vi "0506_Classificador_de_forma.vi"() -> ()   [LabVIEW 2017]
uses:
  <vilib>/userdefined/High Color/IMAQdx.ctl
  <vilib>/vision/driver/IMAQdx.llb/IMAQdx Acquisition Mode.ctl
  <vilib>/vision/driver/IMAQdx.llb/IMAQdx Buffer Number Mode.ctl
  <vilib>/vision/driver/NI_Vision_Acquisition_Software.lvlib
  <vilib>/vision/NI_Vision_Development_Module.lvlib
panel:
  out "size(s)":i32
  out "Forma":string="Quadrado"
  out "Contorno":cluster{"X":dbl, "Y":dbl}[](graph)
  in  "Operation":T1(ring)=enum."Gradient out"
  in  "Convex Hull":bool=TRUE
  in  "Morphology\nOperation":bool
  in  "Remove small objects":bool=TRUE
  in  "Color Mode":u16(ring) items=["RGB", "HSL", "HSV", "HSI"]
  in  "Red or Hue Range":cluster{"Lower value":sgl, "Upper value":sgl}={"Lower value"=0.0, "Upper value"=255.0} {"Upper value" scale=0.0..255.0; "Lower value" scale=0.0..255.0}
  in  "Green or Sat Range":cluster{"Lower value":sgl, "Upper value":sgl}={"Lower value"=0.0, "Upper value"=255.0} {"Upper value" scale=0.0..255.0; "Lower value" scale=0.0..255.0}
  in  "Blue or Luma or Val or Inten Range":cluster{"Lower value":sgl, "Upper value":sgl}={"Lower value"=0.0, "Upper value"=200.09125} {"Upper value" scale=0.0..255.0; "Lower value" scale=0.0..255.0}
  out "Imagem Processada":T2(plugin-control)
  out "Imagem Original":T2(plugin-control)
  in  "Stop Button":bool
  out "dt":dbl
  in  "Câmera":T3="cam1"
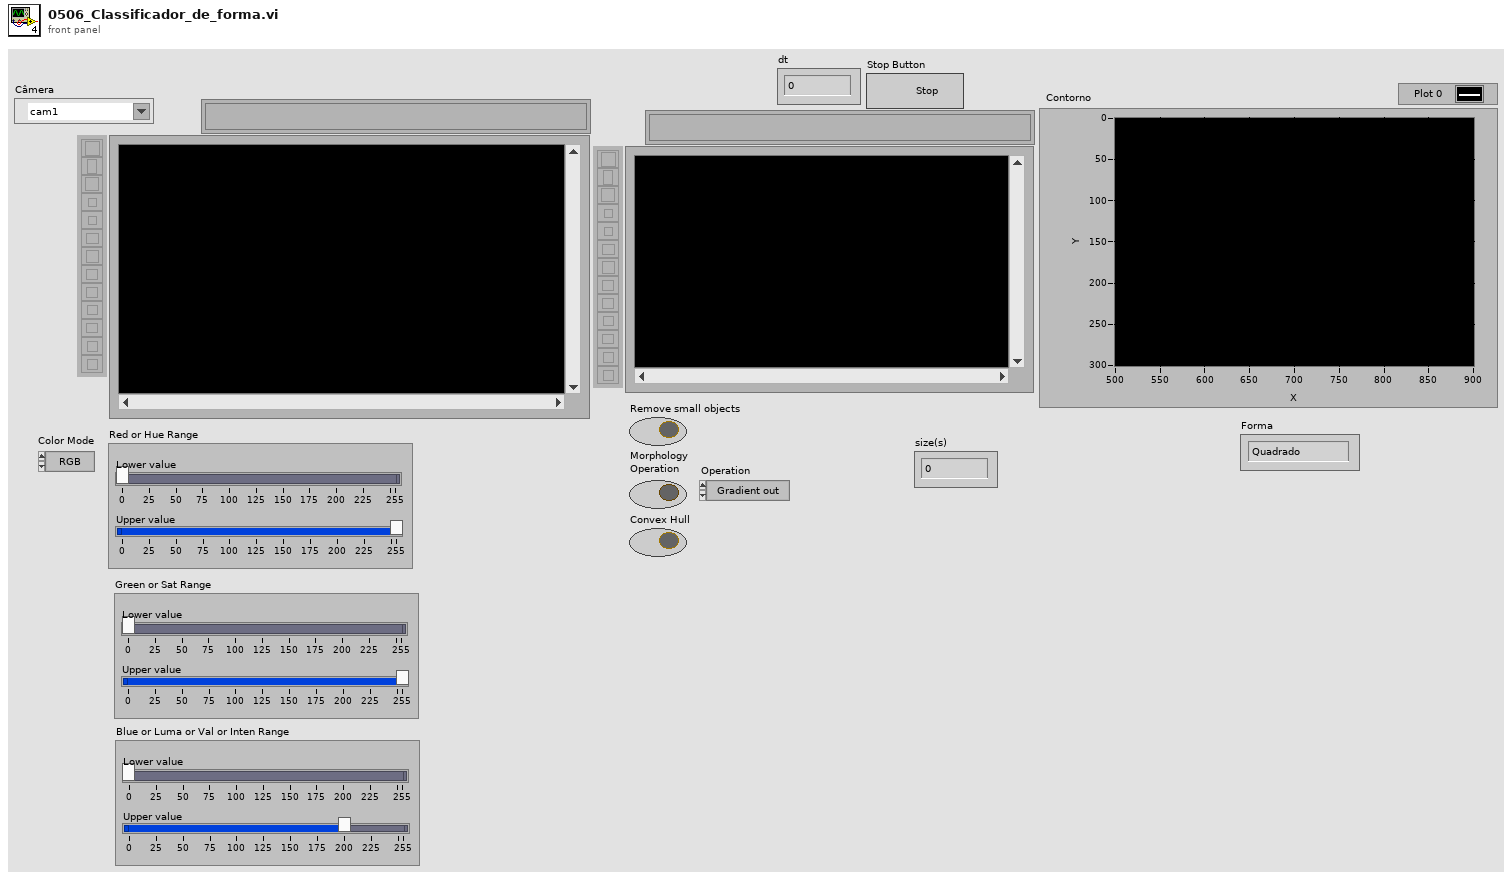
[diagram p1: front panel]
types:
  T1 = enum32{"AutoM", "Close", "Dilate", "Erode", "Gradient", "Gradient out", "Gradient in", "Hit miss", "Open", "PClose", "POpen", "Thick", "Thin"}
  T2 = typedef "IMAQ Image.ctl" = refnum<image>
  T3 = typedef "IMAQdx.ctl" = refnum<k21>
  T4 = typedef "Image Type" = u32
  T5 = typedef "NI_Vision_Acquisition_Software.lvlib/IMAQdx Acquisition Mode.ctl" = enum32{"One Shot", "Continuous"}
  T6 = typedef "NI_Vision_Acquisition_Software.lvlib/IMAQdx Buffer Number Mode.ctl" = enum32{"Next", "Last", "Buffer Number", "Every", "Last New"}
  T7 = cluster{"Global Rectangle":i32[], "Contours":cluster{"Contour Type":u32, "ROI Type":u32, "Points":i32[]}[]}
  T8 = typedef "IMAQ ExtractCurvesCurve.ctl" = cluster{"Points":cluster{"X":dbl, "Y":dbl}[], "Closed?":bool, "Curve Length":dbl, "Min Edge Strength":dbl, "Max Edge Strength":dbl, "Average Edge Strength":dbl}
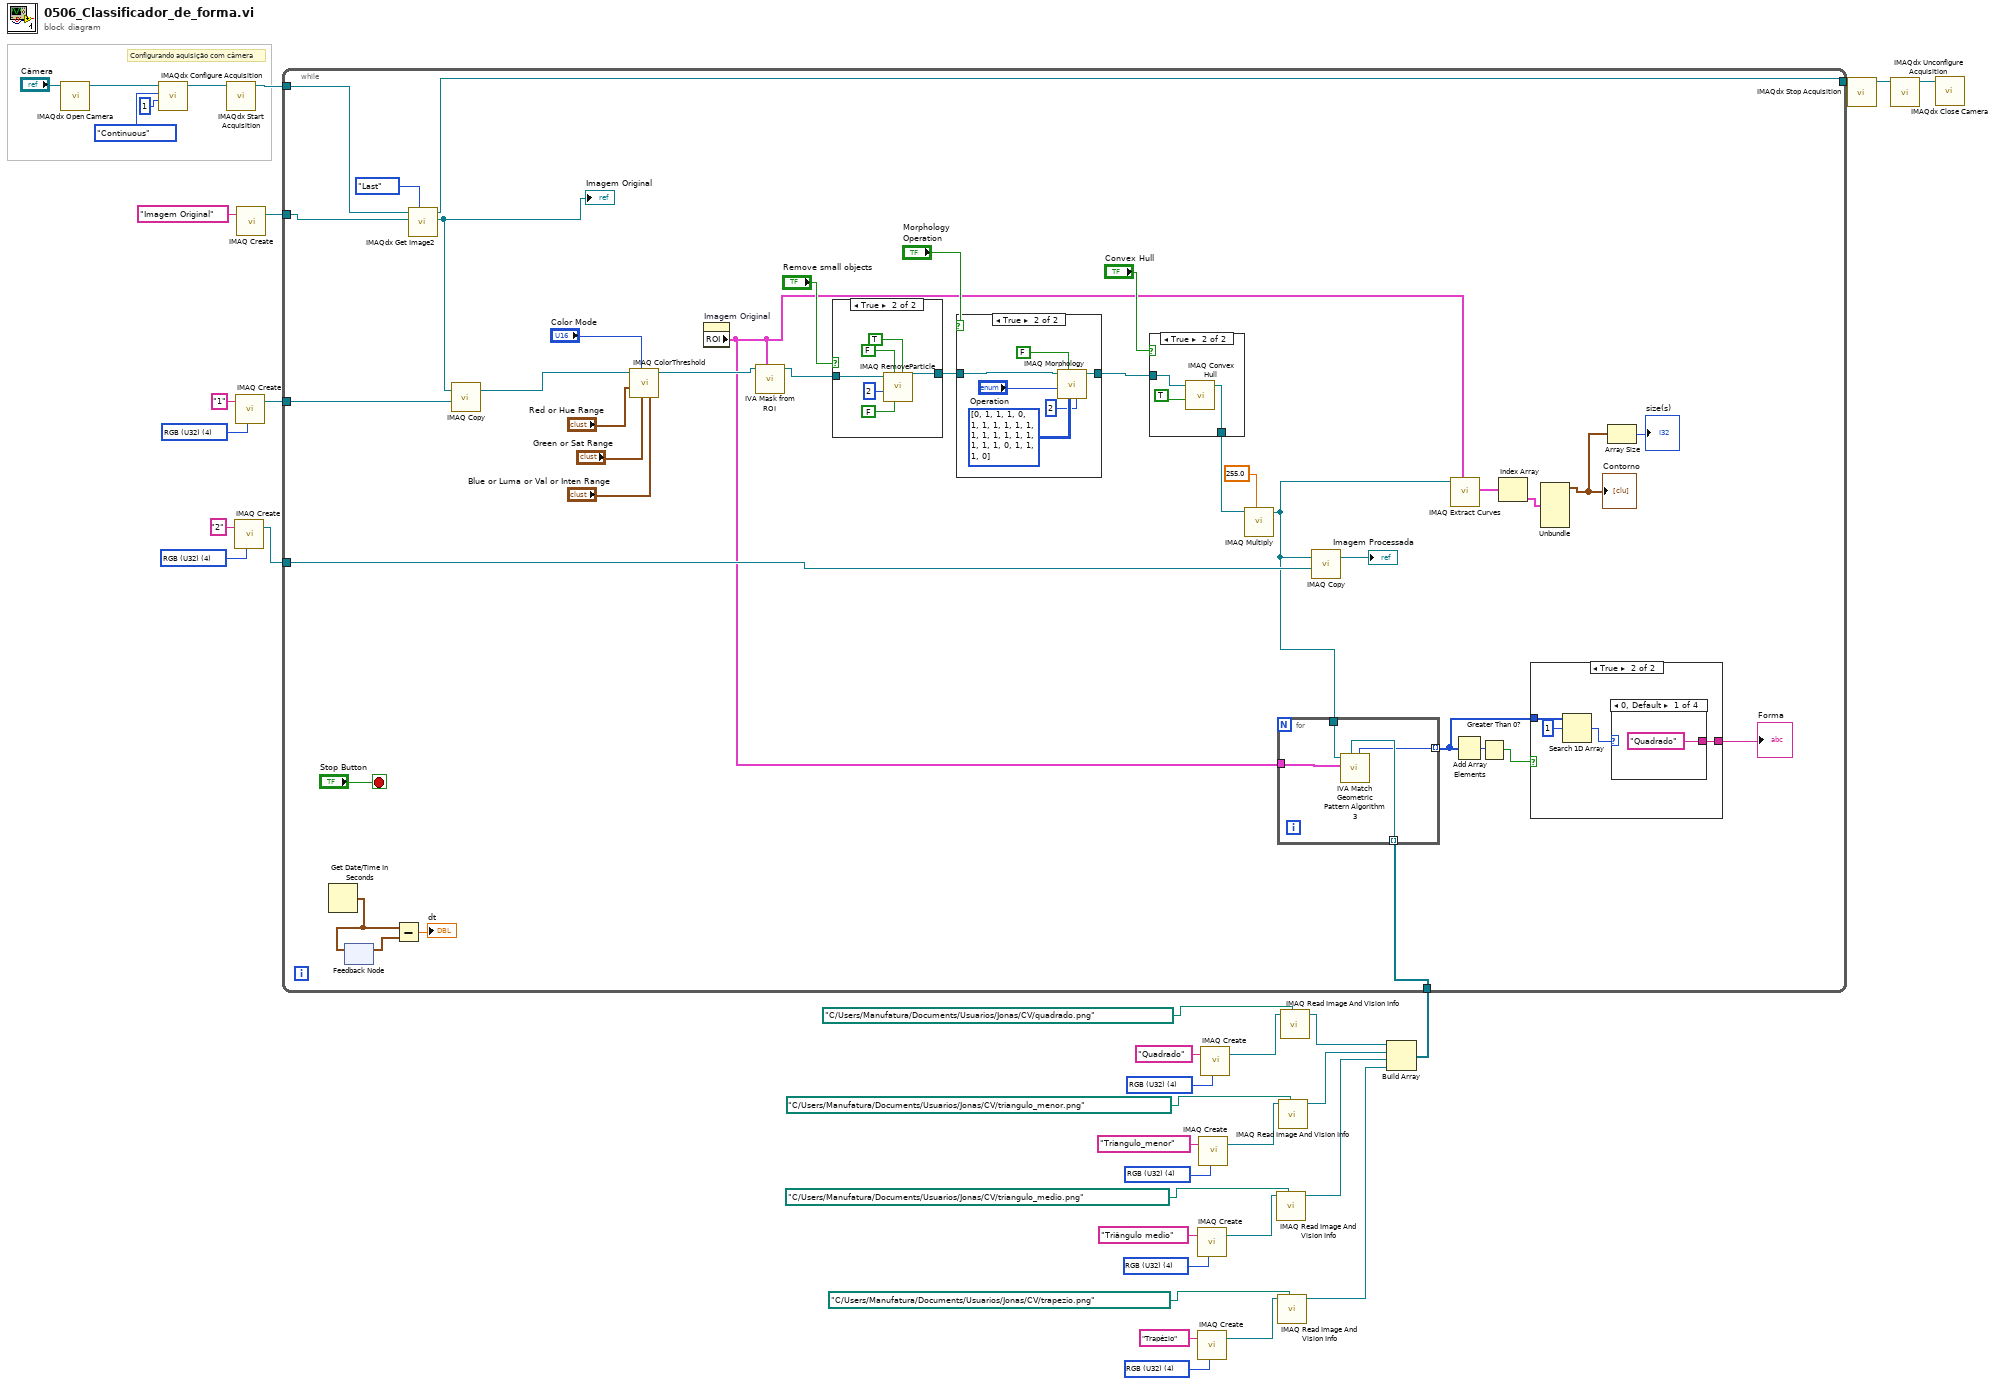
[diagram p0: block diagram]
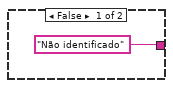
[diagram p2: hidden frame]
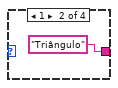
[diagram p3: hidden frame]
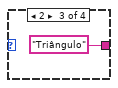
[diagram p4: hidden frame]
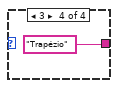
[diagram p5: hidden frame]
diagram:
  w7 = T4 4 items=["Grayscale (U8)", "Grayscale (I16)", "Grayscale (SGL)", "Complex (CSG)", "RGB (U32)", "HSL (U32)", "RGB (U64)", "Grayscale (U16)"] ("Image Type")
  w12 = T4 4 items=["Grayscale (U8)", "Grayscale (I16)", "Grayscale (SGL)", "Complex (CSG)", "RGB (U32)", "HSL (U32)", "RGB (U64)", "Grayscale (U16)"] ("Image Type")
  w15 = T4 4 items=["Grayscale (U8)", "Grayscale (I16)", "Grayscale (SGL)", "Complex (CSG)", "RGB (U32)", "HSL (U32)", "RGB (U64)", "Grayscale (U16)"] ("Image Type")
  w20 = T4 4 items=["Grayscale (U8)", "Grayscale (I16)", "Grayscale (SGL)", "Complex (CSG)", "RGB (U32)", "HSL (U32)", "RGB (U64)", "Grayscale (U16)"] ("Image Type")
  w27 = T4 4 items=["Grayscale (U8)", "Grayscale (I16)", "Grayscale (SGL)", "Complex (CSG)", "RGB (U32)", "HSL (U32)", "RGB (U64)", "Grayscale (U16)"] ("Image Type")
  w29 = T4 4 items=["Grayscale (U8)", "Grayscale (I16)", "Grayscale (SGL)", "Complex (CSG)", "RGB (U32)", "HSL (U32)", "RGB (U64)", "Grayscale (U16)"] ("Image Type")
  # "Configurando aquisição com câmera"
  n1 = call <vilib>:"IMAQdx Open Camera.vi"("Session In"="Câmera") -> ("Session Out"=w38:T3)  [unwired: 9 in, 1 out]
  n2 = call <vilib>:"IMAQdx Configure Acquisition.vi"("Number of Buffers"=u32 1, "Continuous?"=IMAQdx_Acquisition_Mode."Continuous", "Session In"=w38) -> ("Session Out"=w37:T3)  [unwired: 7 in, 1 out]
  n3 = call <vilib>:"IMAQdx Start Acquisition.vi"("Session In"=w37) -> ("Session Out"=w28:T3)  [unwired: 9 in, 1 out]
  n4 = call "IMAQ Create"("Image Name"="2", "Image Type"=w27) -> ("New Image"=w25:T2)  [unwired: 3 in, 1 out]
  n5 = call "IMAQ Create"("Image Name"="1", "Image Type"=w29) -> ("New Image"=w30:T2)  [unwired: 3 in, 1 out]
  n6 = call "IMAQ Create"("Image Name"="Imagem Original") -> ("New Image"=w34:T2)  [unwired: 4 in, 1 out]
  n7 = call "IMAQ Create"("Image Name"="Triângulo medio", "Image Type"=w15) -> ("New Image"=w16:T2)  [unwired: 3 in, 1 out]
  n8 = call "IMAQ Create"("Image Name"="Trapézio", "Image Type"=w12) -> ("New Image"=w11:T2)  [unwired: 3 in, 1 out]
  n9 = call "IMAQ Create"("Image Name"="Triangulo_menor", "Image Type"=w7) -> ("New Image"=w8:T2)  [unwired: 3 in, 1 out]
  n10 = call "IMAQ Create"("Image Name"="Quadrado", "Image Type"=w20) -> ("New Image"=w19:T2)  [unwired: 3 in, 1 out]
  n11 = call "IMAQ Read Image And Vision Info"("File Path"=path "C:/Users/Manufatura/Documents/Usuarios/Jonas/CV/triangulo_medio.png" ("Template File Path"), "Image"=w16) -> ("Image Out"=w3:T2)  [unwired: 2 in, 7 out]
  n12 = call "IMAQ Read Image And Vision Info"("File Path"=path "C:/Users/Manufatura/Documents/Usuarios/Jonas/CV/trapezio.png" ("Template File Path"), "Image"=w11) -> ("Image Out"=w2:T2)  [unwired: 2 in, 7 out]
  n13 = call "IMAQ Read Image And Vision Info"("File Path"=path "C:/Users/Manufatura/Documents/Usuarios/Jonas/CV/triangulo_menor.png" ("Template File Path"), "Image"=w8) -> ("Image Out"=w4:T2)  [unwired: 2 in, 7 out]
  n14 = call "IMAQ Read Image And Vision Info"("File Path"=path "C:/Users/Manufatura/Documents/Usuarios/Jonas/CV/quadrado.png" ("Template File Path"), "Image"=w19) -> ("Image Out"=w5:T2)  [unwired: 2 in, 7 out]
  n15 = Build Array(w5, w4, w3, w2) -> (w1:T2[])
  n16 = while {
    tunnel: w34 -> [w75]
    tunnel: w30 -> [w73]
    tunnel: w28 -> [w72]
    tunnel: [w71] -> w22
    tunnel: w25 -> [w66]
    tunnel: w1 -> [w47]
    stop <- "Stop Button" stop-if-true
    n17 = Get Date/Time In Seconds() -> (seconds since 1Jan1904=w68:timestamp)
    n18 = feedback #1() -> (w70:timestamp)  [unwired: 1 in]
    n19 = feedback-in #1(w68) -> ()
    n20 = Subtract(x=w68, y=w70) -> (x-y=→"dt":dbl)
    n21 = call <vilib>:"IMAQdx Get Image2.vi"("Buffer Number Mode (Next)"=IMAQdx_Buffer_Number_Mode."Last", "Image In"=w75, "Session In"=w72) -> ("Image Out"=w60:T2, "Session Out"=w71:T3)  [unwired: 5 in, 2 out]
    "Imagem Original" <- w60
    n22 = call "IMAQ Copy"("Image Dst"=w73, "Image Src"=w60) -> ("Image Dst Out"=w58:T2)  [unwired: 4 in, 1 out]
    n23 = call "IMAQ ColorThreshold"("Blue or Luma or Val or Inten Range"="Blue or Luma or Val or Inten Range", "Green or Sat Range"="Green or Sat Range", "Color Mode"="Color Mode", "Red or Hue Range"="Red or Hue Range", "Image Src"=w58) -> ("Image Dst Out"=w57:T2)  [unwired: 3 in, 3 out]
    n24 = property on="Imagem Original" class="ImageControl"() -> ("ROI"=w46:T7)  [unwired: 2 in, 2 out]
    n25 = call <vilib>:"IVA Mask from ROI.vi"("ROI Descriptor"=w46, "Image Src"=w57) -> ("Image Out"=w56:T2)  [unwired: 3 in, 6 out]
    n26 = case shown="True" "Remove small objects" {
      tunnel: w56 -> [w100 w102]
      tunnel: [w100 w101] -> w55
      frame False {
      }
      frame True {
        n27 = call "IMAQ RemoveParticle"("Connectivity 4/8 (8)"=TRUE, "Low Pass/High Pass (Low)"=FALSE, "Square/Hexa (Square)"=FALSE, "Number of Erosion"=2, "Image Src"=w102) -> ("Image Dst Out"=w101:T2)  [unwired: 2 in, 4 out]
      }
    }
    n28 = case shown="True" "Morphology\nOperation" {
      tunnel: [w93 w96] -> w59
      tunnel: w55 -> [w93 w95]
      frame False {
      }
      frame True {
        n29 = call "IMAQ Morphology"("Number of iterations (1)"=2, "Structuring Element"=i32[][] [[0, 1, 1, 1, 0], [1, 1, 1, 1, 1], [1, 1, 1, 1, 1], [1, 1, 1, 1, 1], [0, 1, 1, 1, 0]], "Square/Hexa (Square)"=FALSE, "Operation"="Operation", "Image Src"=w95) -> ("Image Dst Out"=w96:T2)  [unwired: 2 in, 4 out]
      }
    }
    n30 = case shown="True" "Convex Hull" {
      tunnel: w59 -> [w89 w91]
      tunnel: [w89 w90] -> w51
      frame False {
      }
      frame True {
        n31 = call "IMAQ Convex Hull"("Connectivity 4/8 (8)"=TRUE, "Image Src"=w91) -> ("Image Dst Out"=w90:T2)  [unwired: 2 in, 7 out]
      }
    }
    n32 = call "IMAQ Multiply"("Image Src A"=w51, "Constant"=255.0) -> ("Image Dst Out"=w45:T2)  [unwired: 5 in, 1 out]
    n33 = for {
      tunnel: w47 -> [w86] mode=indexing
      tunnel: w46 -> [w88]
      tunnel: w45 -> [w87]
      tunnel: [w85] -> w42 mode=indexing
      n34 = call <vilib>:"IVA Match Geometric Pattern Algorithm 3.vi"("Template"=w86, "ROI Descriptor"=w88, "Image"=w87) -> ("Number of Matches"=w85:i32)  [unwired: 2 in, 6 out]
    }
    n35 = call "IMAQ Copy"("Image Dst"=w66, "Image Src"=w45) -> ("Image Dst Out"=→"Imagem Processada":T2)  [unwired: 4 in, 1 out]
    n36 = call "IMAQ Extract Curves"("ROI Descriptor"=w46, "Image"=w45) -> ("Curves"=w49:T8[])  [unwired: 7 in, 2 out]
    n37 = Add Array Elements(numeric array=w42) -> (sum=w44:i32)
    n38 = Greater Than 0?(x=w44) -> (x > 0?=w43:bool)
    n39 = Index Array(array=w49) -> (element=w48:T8)  [unwired: 1 in]
    n40 = case shown="True" w43 {
      tunnel: w42 -> [_ w80]
      tunnel: ["Não identificado" w77] -> w41
      frame False {
      }
      frame True {
        n41 = Search 1D Array(1D array=w80, element=1) -> (index of element=w78:i32)  [unwired: 1 in]
        n42 = case shown="0, Default" w78 {
          tunnel: ["Quadrado" "Triângulo" "Triângulo" "Trapézio"] -> w77
          frame 0, Default {
          }
          frame 1 {
          }
          frame 2 {
          }
          frame 3 {
          }
        }
      }
    }
    "Forma" <- w41
    n43 = Unbundle(w48) -> ("Points"=w40:cluster{"X":dbl, "Y":dbl}[])  [unwired: 5 out]
    "Contorno" <- w40
    n44 = Array Size(array=w40) -> (size(s)=→"size(s)":i32)
  }
  n45 = call <vilib>:"IMAQdx Stop Acquisition.vi"("Session In"=w22) -> ("Session Out"=w24:T3)  [unwired: 9 in, 1 out]
  n46 = call <vilib>:"IMAQdx Unconfigure Acquisition.vi"("Session In"=w24) -> ("Session Out"=w23:T3)  [unwired: 9 in, 1 out]
  n47 = call <vilib>:"IMAQdx Close Camera.vi"("Session In"=w23) -> ()  [unwired: 10 in, 1 out]
